vi "geo-tsk1.vi"() -> ()   [LabVIEW 2020]
panel:
  out "nth sum":dbl
  out "nth element":dbl
  in  "n":dbl
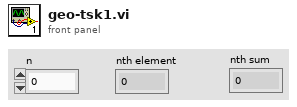
[diagram p1: front panel]
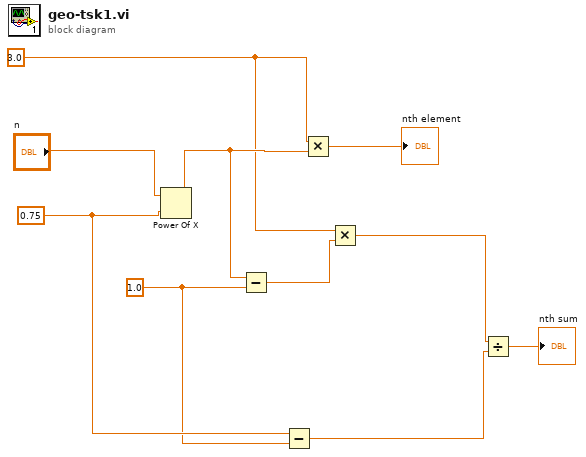
[diagram p0: block diagram]
diagram:
  w4 = 1.0
  w5 = 0.75
  w7 = 3.0
  n1 = Power Of X(1:w5, 2:"n") -> (0:w8:dbl)
  n2 = Subtract(x=w8, y=w4) -> (x-y=w6:dbl)
  n3 = Subtract(x=w5, y=w4) -> (x-y=w2:dbl)
  n4 = Multiply(x=w7, y=w8) -> (x*y=→"nth element":dbl)
  n5 = Multiply(x=w7, y=w6) -> (x*y=w3:dbl)
  n6 = Divide(x=w3, y=w2) -> (x/y=→"nth sum":dbl)
